vi "Init.vi"(8 "error in (no error)":errorcluster, 11 "RealSubject2 in":refnum<class "RealSubject2.lvclass">) -> (0 "error out":errorcluster, 3 "RealSubject2 out":refnum<class "RealSubject2.lvclass">)   [LabVIEW 2014, in "Normal Proxy.lvlib" / "RealSubject2.lvclass"]
uses:
  RealSubject2.lvclass
  Subject/Subject.lvclass/Subject.ctl
  Subject/Subject.lvclass
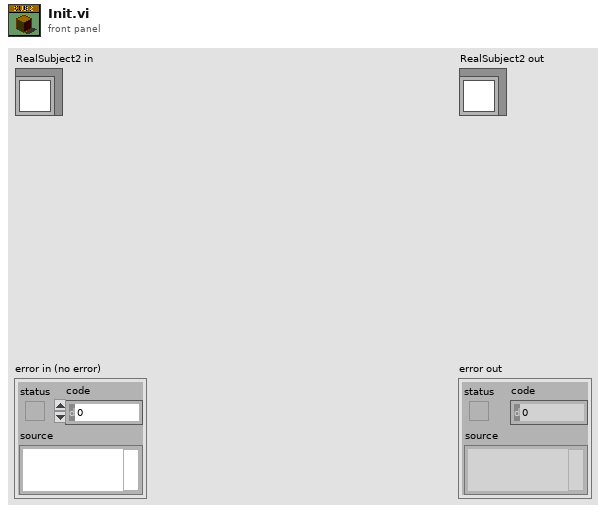
[diagram p1: front panel]
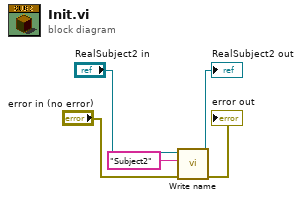
[diagram p0: block diagram]
diagram:
  n1 = call "Write name.vi"("error in (no error)"="error in (no error)", "name"="Subject2", "Subject in"="RealSubject2 in") -> ("error out"=→"error out":errorcluster, "Subject out"=→"RealSubject2 out":refnum<class "RealSubject2.lvclass">)  [unwired: 7 in]
